vi "Some String Inside 2.vi"(8 "Error In":errorcluster) -> (0 "Error Out":errorcluster)   [LabVIEW 2018]
uses:
  <vilib>/measure/NI_MABase.lvlib
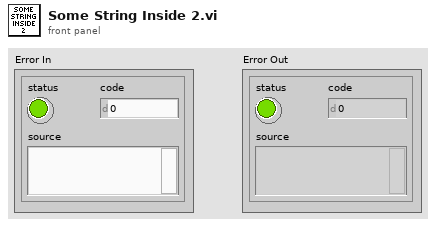
[diagram p1: front panel]
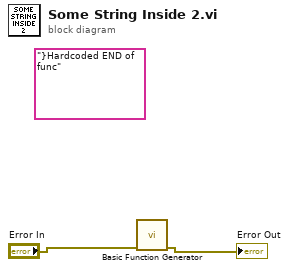
[diagram p0: block diagram]
diagram:
  (unwired) "}Hardcoded END of func"
  n1 = call <vilib>:"Basic Function Generator.vi"("error in (no error)"="Error In") -> ("error out"=→"Error Out":errorcluster)  [unwired: 8 in, 2 out]
